vi "test_AM_PID.vi"() -> ()   [LabVIEW 2013]
uses:
  <vilib>/rvi/FXPMathLib/FxpConvert/subVIs/nifxpmath_Convert_SimConfig.ctl
  <vilib>/fxp/LVFixedPointQuantizationPolicyTypeDef.ctl
  <vilib>/fxp/LVFixedPointOverflowPolicyTypeDef.ctl
  <vilib>/rvi/FXPMathLib/FxpConvert/simVIs/DllFxpConvertTemp_sub.vi
  <vilib>/rvi/FXPMathLib/FxpConvert/XNode/nifxpmath_Convert.xnode
  <vilib>/measure/NI_MABase.lvlib
panel:
  out "size(s)":i32
  out "Waveform Graph 4":i16[](graph)
  out "Waveform Graph 3":dbl[][](graph)
  out "Waveform Graph":dbl[](graph)
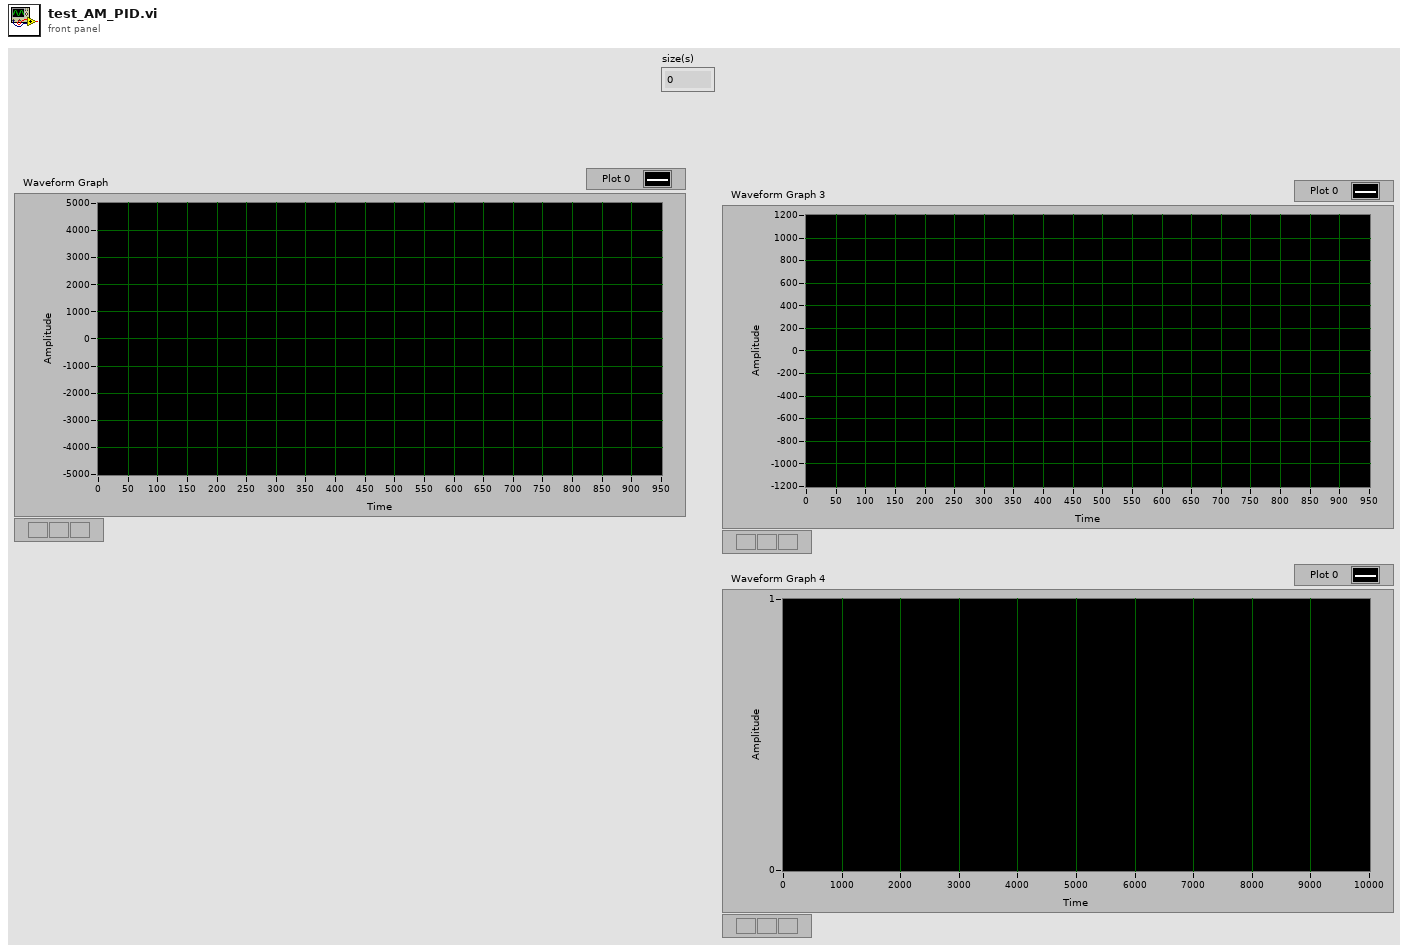
[diagram p1: front panel]
types:
  T1 = cluster{"frequency":dbl, "amplitude":dbl, "phase":dbl}[]
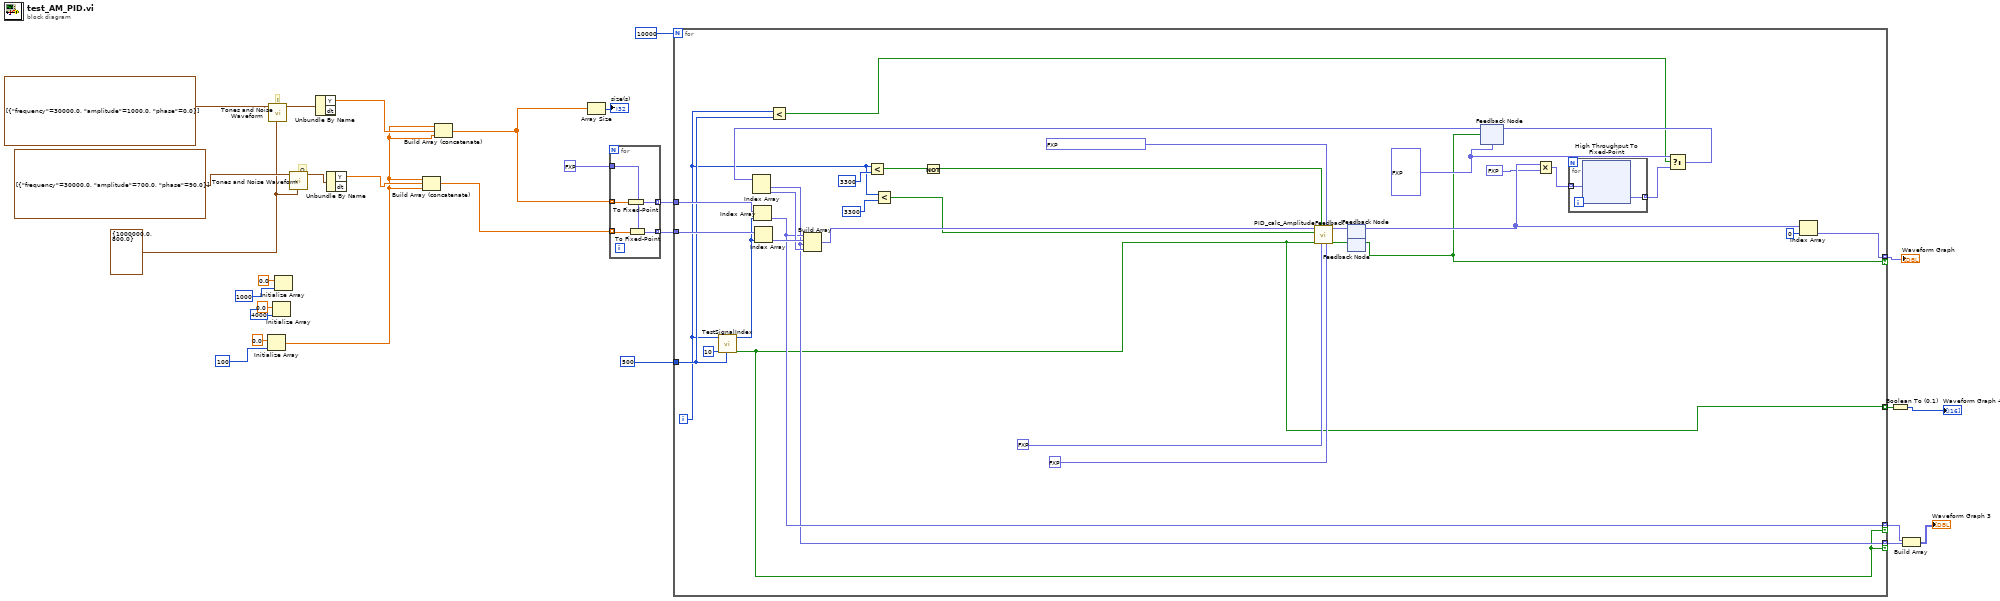
[diagram p0: block diagram]
diagram:
  w23 = cluster{"Fs":dbl, "#s":dbl} {"Fs"=1000000.0, "#s"=800.0} ("sampling info")
  # "Q"
  # "I"
  n1 = Initialize Array(0.0 ("element"), 100 ("dimension size")) -> (w13:dbl[])
  n2 = call <vilib>:"Tones and Noise Waveform.vi"("sampling info"=w23, "tones"=T1 [{"frequency"=30000.0, "amplitude"=1000.0, "phase"=0.0}]) -> ("signal out"=w26:waveform(dbl))  [unwired: 8 in, 1 out]
  n3 = Initialize Array(0.0 ("element"), 4000 ("dimension size")) -> ()  [unwired: 1 out]
  n4 = Initialize Array(0.0 ("element"), 1000 ("dimension size")) -> ()  [unwired: 1 out]
  n5 = call <vilib>:"Tones and Noise Waveform.vi"("sampling info"=w23, "tones"=T1 [{"frequency"=30000.0, "amplitude"=700.0, "phase"=90.0}]) -> ("signal out"=w20:waveform(dbl))  [unwired: 8 in, 1 out]
  n6 = Unbundle By Name(w26) -> ("Y"=w16:dbl[])  [unwired: 1 out]
  n7 = Unbundle By Name(w20) -> ("Y"=w15:dbl[])  [unwired: 1 out]
  n8 = Build Array (concatenate)(w13, w15, w13) -> (w12:dbl[])
  n9 = Build Array (concatenate)(w13, w16, w13) -> (w5:dbl[])
  n10 = Array Size(array=w5) -> (size(s)=→"size(s)":i32)
  n11 = for {
    tunnel: w12 -> [w32] mode=indexing
    tunnel: fxp<+/-,16,14> 0.0 ("fixed-point type") -> [w33]
    tunnel: [w31] -> w25 mode=indexing
    tunnel: w5 -> [w29] mode=indexing
    tunnel: [w30] -> w11 mode=indexing
    n12 = To Fixed-Point(number=w29) -> (fixed-point=w30:fxp<+/-,16,14>)  [unwired: 1 in]
    n13 = To Fixed-Point(fixed-point type=w33, number=w32) -> (fixed-point=w31:fxp<+/-,16,14>)
  }
  n14 = for {
    N: 10000 -> [_]
    tunnel: w25 -> [w65]
    tunnel: [w50] -> w7 mode=indexing if=w48
    tunnel: w11 -> [w64]
    tunnel: [w38] -> w3 mode=indexing if=w36
    tunnel: [w36] -> w9 mode=indexing
    tunnel: 500 ("initial delay") -> [w52]
    tunnel: [w37] -> w2 mode=indexing if=w36
    i -> [w40]
    w59 = fxp<+/-,16,14>[] [0.0, 0.0]
    n15 = call "TestSignalIndex.vi"("initial delay"=w52, "cycles per sample"=10, "index"=w40) -> ("valid out"=w36:bool, "array index"=w61:i32)  [unwired: 7 in]
    n16 = Index Array(array=w64, index=w61) -> (element=w38:fxp<+/-,16,14>)
    n17 = Index Array(array=w65, index=w61) -> (element=w62:fxp<+/-,16,14>)
    n18 = Less?(x=w40, y=w52) -> (x < y?=w53:bool)
    n19 = Less?(x=w40, y=3300 ("initial delay")) -> (x < y?=w35:bool)
    n20 = Less?(x=w40, y=3300 ("initial delay")) -> (x < y?=w34:bool)
    n21 = Not(x=w35) -> (.not. x?=w41:bool)
    n22 = feedback #1() -> (w51:fxp<+/-,16,14>[])  [unwired: 1 in]
    n23 = feedback #2() -> (w48:bool)  [unwired: 1 in]
    n24 = feedback #3(w59) -> (w63:fxp<+/-,16,14>[])
    n25 = Index Array(array=w63) -> (element #1=w37:fxp<+/-,16,14>, element #2=w43:fxp<+/-,16,14>)  [unwired: 2 in]
    n26 = Build Array(w38, w62, w37, w43) -> (w54:fxp<+/-,16,14>[])
    n27 = call "PID_calc_AmplitudeFeedback.vi"("Kd/Tau"=fxp<+/-,32,6> 0.0 ("Data"), "Ki*Tau"=fxp<+/-,32,6> 0.0010000020265579224 ("Data"), "Kp"=fxp<+/-,32,6> 0.0 ("Data"), "Enabled"=w41, "input valid"=w36, "Reset"=w34, "Data in"=w54) -> ("output valid"=w49:bool, "data out"=w58:fxp<+/-,16,14>[])  [unwired: 1 in, 2 out]
    n28 = feedback-in #1(w58) -> ()
    n29 = feedback-in #2(w49) -> ()
    n30 = Multiply(x=w51, y=fxp<+,1,-1> 0.25 ("x*y")) -> (x*y=w45:fxp<+/-,16,12>[])
    n31 = for {
      tunnel: w45 -> [w68] mode=indexing
      tunnel: [w67] -> w44 mode=indexing
      n32 = xnode "High Throughput To Fixed-Point"("x"=w68) -> ("y"=w67:fxp<+/-,16,14>)
    }
    n33 = Select(t=w59, s=w53, f=w44) -> (s? t:f=w60:fxp<+/-,16,14>[])
    n34 = feedback-in #3(w60, w48) -> ()
    n35 = Index Array(array=w51, index=0) -> (element=w50:fxp<+/-,16,14>)
  }
  "Waveform Graph" <- w7
  n36 = Boolean To (0,1)(Boolean=w9) -> (0, 1=→"Waveform Graph 4":i16[])
  n37 = Build Array(w3, w2) -> (→"Waveform Graph 3":fxp<+/-,16,14>[][])
